vi "BoxGlobals.vi"() -> ()   [LabVIEW 2023]
uses:
  BoxNoteState.ctl
panel:
  in  "IntakeGetNoteMotorDMD":dbl=0.5
  in  "ShooterSpeedRPM":dbl=4000.0
  in  "Box Note State":T1
  out "ReadyForCommand":bool
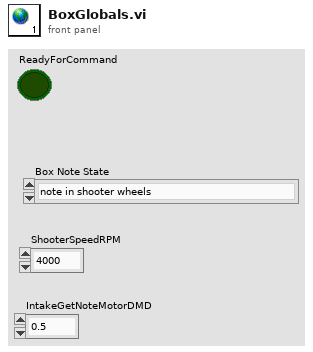
[diagram p1: front panel]
types:
  T1 = typedef "BoxNoteState.ctl" = enum16{"note in shooter wheels", "misaligned note", "no note", "have note"}
diagram:
